vi "Configure Sampling.vi"(8 "error in (no error)":errorcluster, 9 "RIS Mode (F: Off)":bool, 10 "Combine Channels Mode (0: Auto)":u16(ring) items=["Auto", "4", "2"], 11 "VISA resource name":refnum<visa-resource-name>) -> (0 "error out":errorcluster, 3 "VISA resource name out":refnum<visa-resource-name>)   [LabVIEW 2013, in "LeCroy Wave Series.lvlib"]
doc: "Controls the channel interleaving function of the acquisition system and enable or disable RIS mode.\n\nNote:\nThis VI has been obsoleted from the driver and is included for compatibility with existing applications. New applications should use the Configure Sample Mode."
uses:
  LeCroy Wave Series.lvlib
panel:
  # "Note:\nThis VI has been obsoleted from the driver and is included for compatibility with existing applications.  New applications should use the Configure Sample Mode."
  # "T: On\n\nF: Off"
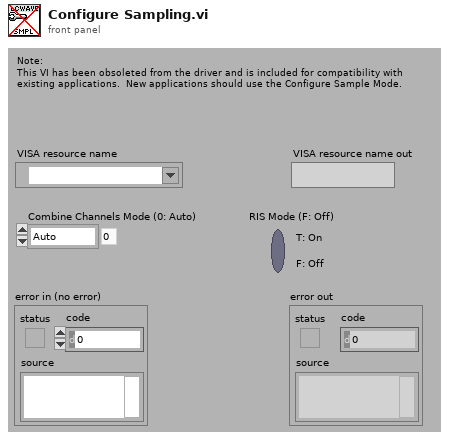
[diagram p1: front panel]
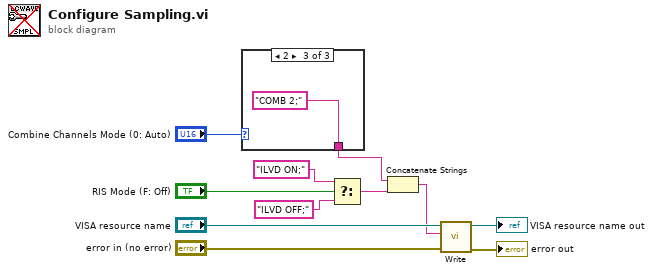
[diagram p0: block diagram]
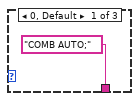
[diagram p2: hidden frame]
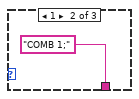
[diagram p3: hidden frame]
diagram:
  n1 = case shown="2" "Combine Channels Mode (0: Auto)" {
    tunnel: ["COMB AUTO;" "COMB 1;" "COMB 2;"] -> w6
    frame 0, Default {
    }
    frame 1 {
    }
    frame 2 {
    }
  }
  n2 = Select(t="ILVD ON;", s="RIS Mode (F: Off)", f="ILVD OFF;") -> (s? t:f=w2:string)
  n3 = Concatenate Strings(w6, w2) -> (w1:string)
  n4 = call "Write.vi"("error in (no error)"="error in (no error)", "Write Buffer"=w1, "VISA resource name"="VISA resource name") -> ("error out"=→"error out":errorcluster, "VISA resource name out"=→"VISA resource name out":refnum<visa-resource-name>)  [unwired: 6 in, 1 out]
